vi "Bank Connection Page.vi"(8 "error in (no error)":errorcluster, 11 "Node Ptr":T1 format="%.0x") -> (0 "error out":errorcluster)   [LabVIEW 2011, in "NI 272x Resistive Simulation Custom Device Configuration.lvlib"]
uses:
  NI 272x Resistive Simulation Custom Device Configuration.lvlib
  <vilib>/NI Veristand/Custom Device API/Custom Device Item Ref.ctl
  Globals/Names.vi
  <vilib>/NI Veristand/Custom Device API/Get Item Property (I32).vi
  <vilib>/NI Veristand/Custom Device API/Set Item Property (I32).vi
  <vilib>/NI Veristand/Custom Device API/Custom Device API.lvlib
  NI 272x Resistive Simulation Custom Device Shared.lvlib
panel:
  out "Adjacent Channel #":i32
  in  "Default Value":dbl
  in  "Channel #":i32 min=0
  in  "Header":cluster{"Section Name":string}={"Section Name"="Bank Connection Setting"}
  in  "Description":string
  in  "Name":string
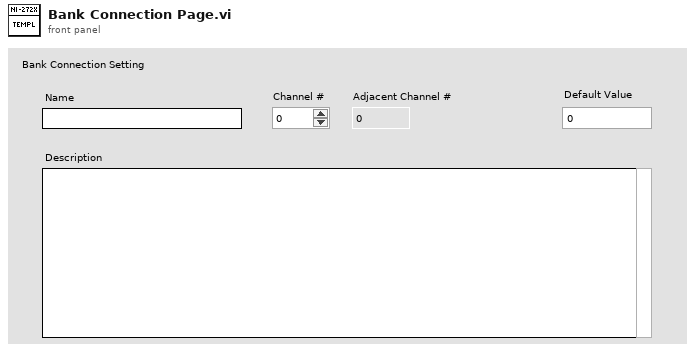
[diagram p1: front panel]
types:
  T1 = typedef "Custom Device API.lvlib/Custom Device Item Ref.ctl" = u64
  T2 = typedef "Custom Device API.lvlib/Custom Device Channel.ctl" = cluster{"Type":T3, "Units":string, "Default Value":dbl, "Faultable":bool, "Scalable":bool}
  T3 = typedef "Custom Device API.lvlib/Custom Device Channel Type.ctl" = enum16{"Input", "Output"}
  T4 = typedef "Custom Device API.lvlib/Custom Device Item Info.ctl" = cluster{"Name":string, "Is Channel":bool, "GUID":string}
  T5 = typedef "Custom Device API.lvlib/Custom Device Commands.ctl" = enum16{"Default", "Item renamed", "Shutdown", "Dynamic button pressed"}
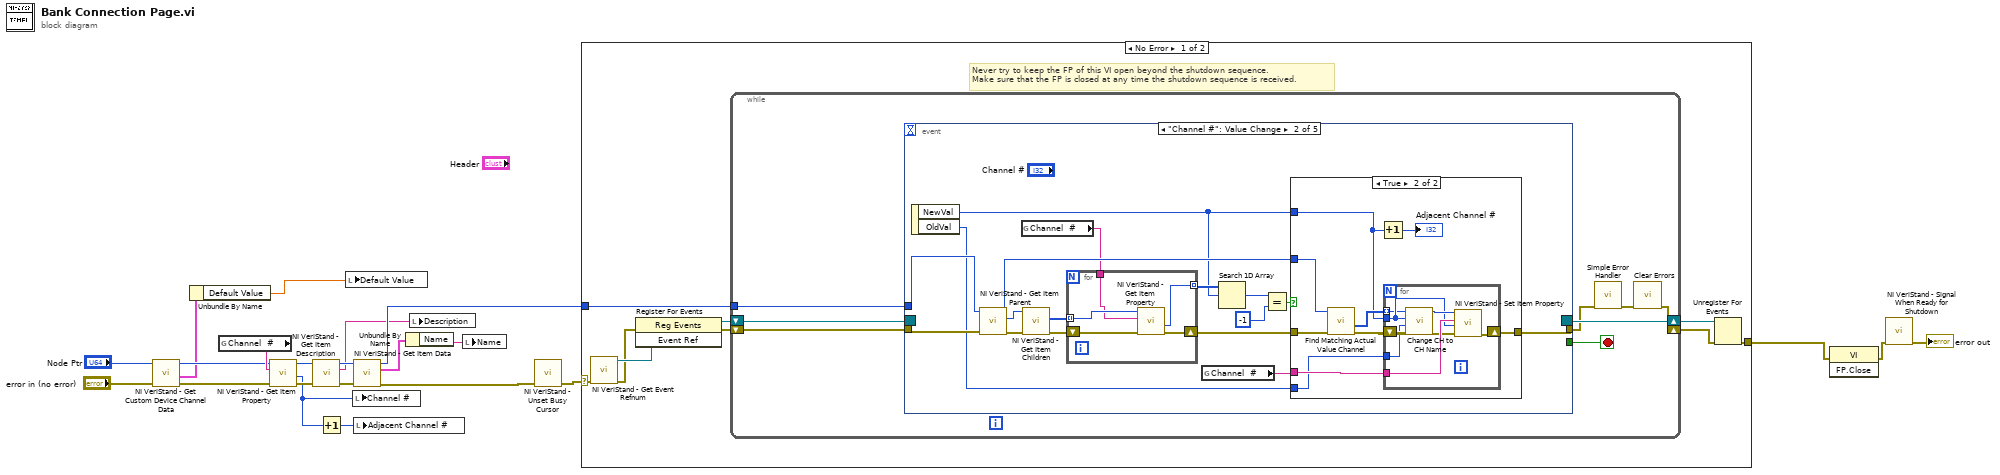
[diagram p0: block diagram]
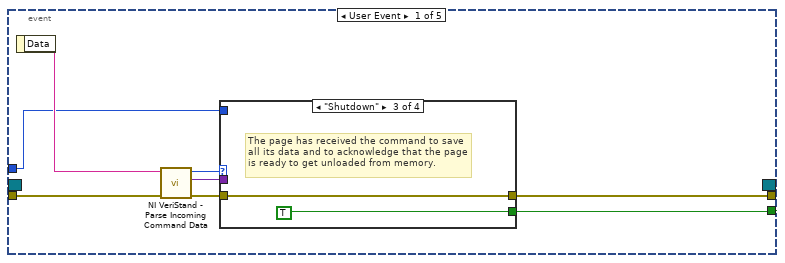
[diagram p2: hidden frame]
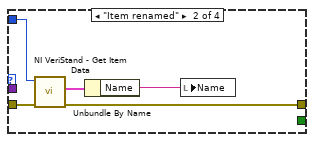
[diagram p4: hidden frame]
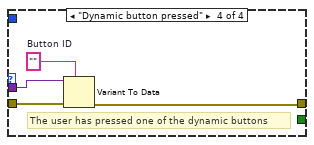
[diagram p5: hidden frame]
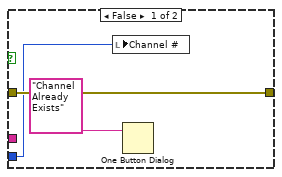
[diagram p6: hidden frame]
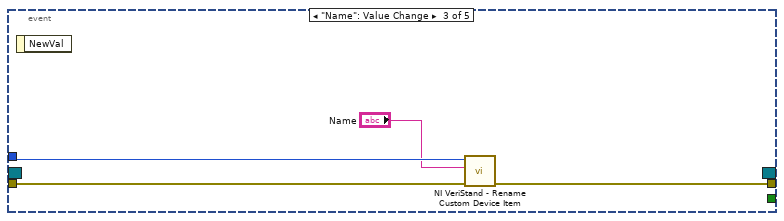
[diagram p7: hidden frame]
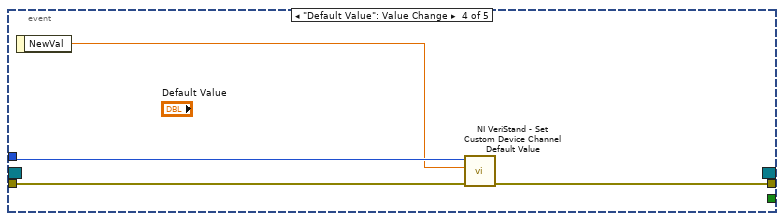
[diagram p8: hidden frame]
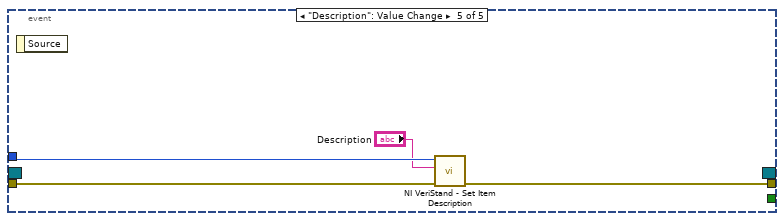
[diagram p9: hidden frame]
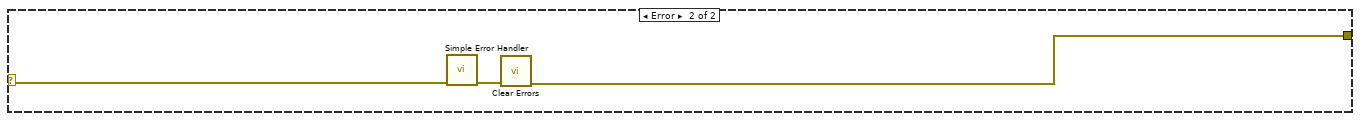
[diagram p10: hidden frame]
diagram:
  n1 = call <vilib>:"NI VeriStand - Get Custom Device Channel Data.vi"("error in (no error)"="error in (no error)", "Channel Ref in"="Node Ptr") -> ("error out"=w5:errorcluster, "Channel"=w2:T2, "Channel Ref out"=w3:T1)  [unwired: 4 in, 3 out]
  n2 = Unbundle By Name(w2) -> ("Default Value"=w1:dbl)
  n3 = global read "Names.vi" "Channel  #"() -> (w9:string)
  n4 = call-poly <vilib>:"NI VeriStand - Get Item Property.vi"("error in (no error)"=w5, "Property Name"=w9, "Item Ref in"=w3) -> ("error out"=w10:errorcluster, "Value"=w7:i32, "Item Ref out"=w11:T1)  [unwired: 5 in, 1 out]
  n5 = call <vilib>:"NI VeriStand - Get Item Description.vi"("error in (no error)"=w10, "Item Ref in"=w11) -> ("error out"=w14:errorcluster, "Description"=w15:string, "Item Ref out"=w16:T1)  [unwired: 7 out]
  n6 = Increment(x=w7) -> (x+1=w6:i32)
  n7 = local write "Default Value"(w1) -> ()
  n8 = local write "Channel #"(w7) -> ()
  n9 = call <vilib>:"NI VeriStand - Get Item Data.vi"("error in (no error)"=w14, "Item Ref in"=w16) -> ("error out"=w8:errorcluster, "Item Info"=w13:T4, "Item Ref out"=w18:T1)  [unwired: 7 out]
  n10 = local write "Adjacent Channel #"(w6) -> ()
  n11 = Unbundle By Name(w13) -> ("Name"=w12:string)
  n12 = local write "Description"(w15) -> ()
  n13 = local write "Name"(w12) -> ()
  n14 = call <vilib>:"NI VeriStand - Unset Busy Cursor.vi"("error in (no error)"=w8) -> ("error out"=w19:errorcluster)  [unwired: 10 out]
  n15 = case shown="No Error" w19 {
    selector: w19 -> [w24 w116]
    tunnel: [w29 w114] -> w22
    tunnel: w18 -> [w25 _]
    frame No Error {
      # "Never try to keep the FP of this VI open beyond the shutdown sequence.\nMake sure that the FP is closed at any time the shutdown sequence is received."
      n16 = call <vilib>:"NI VeriStand - Get Event Refnum.vi"("error in (no error)"=w24) -> ("error out"=w23:errorcluster, "Event Ref"=w28:refnum<user-event>)  [unwired: 9 out]
      n17 = register-events(error in=w23, w28) -> (reference out=w26:refnum<event-registration>, error out=w27:errorcluster)  [unwired: 1 in]
      n18 = while {
        tunnel: w25 -> [w35]
        shift-right: [w33] -> w30
        shift-left: w27 -> [w38]
        shift-right: [w39] -> w31
        shift-left: w26 -> [w37]
        stop <- w36 stop-if-true
        n19 = event shown="[1] \"Channel #\": Value Change" {
          selector: w37 -> [_ _ _ _ _]
          dyn-events: [_ _ _ _ _] -> w39
          timeout: _ -> [_ _ _ _ _]
          tunnel: w38 -> [w47 w66 w105 w109 w112]
          tunnel: [w43 _ _ _ _] -> w36
          tunnel: [w42 w62 w102 w107 w111] -> w32
          tunnel: w35 -> [w41 w65 w104 w108 w113]
          event User Event {
            n20 = event-data() -> ("Data"=w46:string)  [unwired: 1 out]
            n21 = call <vilib>:"NI VeriStand - Parse Incoming Command Data.vi"("error in (no error)"=w47, "Incoming data"=w46) -> ("error out"=w45:errorcluster, "Outgoing data"=w40:variant, "Action"=w44:T5)  [unwired: 7 out]
            n22 = case shown="\"Shutdown\"" w44 {
              tunnel: w45 -> [w48 w53 w54 w59]
              tunnel: [_ _ TRUE _] -> w43
              tunnel: [w48 w50 w54 w56] -> w42
              tunnel: w41 -> [_ w52 _ _]
              tunnel: w40 -> [_ _ _ w58]
              frame "Default", Default {
              }
              frame "Item renamed" {
                n23 = call <vilib>:"NI VeriStand - Get Item Data.vi"("error in (no error)"=w53, "Item Ref in"=w52) -> ("error out"=w50:errorcluster, "Item Info"=w51:T4)  [unwired: 8 out]
                n24 = Unbundle By Name(w51) -> ("Name"=w49:string)
                n25 = local write "Name"(w49) -> ()
              }
              frame "Shutdown" {
                # "The page has received the command to save all its data and to acknowledge that the page is ready to get unloaded from memory."
              }
              frame "Dynamic button pressed" {
                w57 = ""  # Button ID
                # "The user has pressed one of the dynamic buttons"
                n26 = Variant To Data(error in=w59, type=w57, Variant=w58) -> (error out=w56:errorcluster)  [unwired: 1 out]
              }
            }
          }
          event "Channel #": Value Change {
            n27 = event-data() -> ("NewVal"=w64:i32, "OldVal"=w63:i32)  [unwired: 1 out]
            n28 = call <vilib>:"NI VeriStand - Get Item Parent.vi"("error in (no error)"=w66, "Item Ref in"=w65) -> ("error out"=w67:errorcluster, "Parent Ref"=w68:T1, "Item Ref out"=w76:T1)  [unwired: 6 in, 1 out]
            n29 = global read "Names.vi" "Channel  #"() -> (w60:string)
            n30 = call <vilib>:"NI VeriStand - Get Item Children.vi"("error in (no error)"=w67, "Item Ref in"=w68) -> ("error out"=w70:errorcluster, "Child Refs"=w69:T1[])  [unwired: 6 in, 2 out]
            n31 = for {
              tunnel: w69 -> [w99] mode=indexing
              shift-right: [w100] -> w75
              shift-left: w70 -> [w101]
              tunnel: [w98] -> w71 mode=indexing
              tunnel: w60 -> [w97]
              n32 = call-poly <vilib>:"NI VeriStand - Get Item Property.vi"("error in (no error)"=w101, "Property Name"=w97, "Item Ref in"=w99) -> ("error out"=w100:errorcluster, "Value"=w98:i32)  [unwired: 5 in, 2 out]
            }
            n33 = global read "Names.vi" "Channel  #"() -> (w61:string)
            n34 = Search 1D Array(1D array=w71, element=w64) -> (index of element=w72:i32)  [unwired: 1 in]
            n35 = Equal?(x=w72, y=-1) -> (x = y?=w74:bool)
            n36 = case shown="True" w74 {
              tunnel: w75 -> [w79 w86]
              tunnel: w76 -> [_ w85]
              tunnel: w61 -> [_ w87]
              tunnel: w64 -> [_ w81]
              tunnel: [w79 w88] -> w62
              tunnel: w63 -> [w77 w82]
              frame False {
                n37 = local write "Channel #"(w77) -> ()
                n38 = One Button Dialog(message="Channel Already Exists") -> ()  [unwired: 1 in, 1 out]
              }
              frame True {
                n39 = call "Find Matching Actual Value Channel.vi"("error in (no error)"=w86, "Desired item ref in"=w85) -> ("error out"=w84:errorcluster, "Both refs"=w83:T1[])  [unwired: 5 in, 3 out]
                n40 = Increment(x=w81) -> (x+1=→"Adjacent Channel #":i32)
                n41 = for {
                  tunnel: w87 -> [w95]
                  shift-right: [w96] -> w88
                  shift-left: w84 -> [w93]
                  tunnel: w81 -> [w91]
                  tunnel: w83 -> [w90] mode=indexing
                  tunnel: w82 -> [w89]
                  n42 = call "Change CH to CH Name.vi"("error in (no error)"=w93, "Old #"=w89, "New #"=w91, "Node Ptr"=w90) -> ("error out"=w94:errorcluster, "Node Ptr out"=w92:T1)  [unwired: 6 in]
                  n43 = call-poly <vilib>:"NI VeriStand - Set Item Property.vi"("error in (no error)"=w94, "Value"=w91, "Property Name"=w95, "Item Ref in"=w92) -> ("error out"=w96:errorcluster)  [unwired: 5 in, 2 out]
                }
              }
            }
          }
          event "Name": Value Change {
            n44 = event-data() -> ()  [unwired: 2 out]
            n45 = call <vilib>:"NI VeriStand - Rename Custom Device Item.vi"("error in (no error)"=w105, "New Name"="Name", "Item Ref in"=w104) -> ("error out"=w102:errorcluster)  [unwired: 8 out]
          }
          event "Default Value": Value Change {
            n46 = event-data() -> ("NewVal"=w106:dbl)  [unwired: 1 out]
            n47 = call <vilib>:"NI VeriStand - Set Custom Device Channel Default Value.vi"("error in (no error)"=w109, "Default Value"=w106, "Channel Ref in"=w108) -> ("error out"=w107:errorcluster)  [unwired: 7 in, 1 out]
          }
          event "Description": Value Change {
            n48 = event-data() -> ()  [unwired: 2 out]
            n49 = call <vilib>:"NI VeriStand - Set Item Description.vi"("error in (no error)"=w112, "Description"="Description", "Item Ref in"=w113) -> ("error out"=w111:errorcluster)  [unwired: 8 out]
          }
        }
        n50 = call <vilib>:"Simple Error Handler.vi"("error in (no error)"=w32) -> ("error out"=w34:errorcluster)  [unwired: 1 in, 7 out]
        n51 = call <vilib>:"Clear Errors.vi"("error in (no error)"=w34) -> ("error out"=w33:errorcluster)  [unwired: 6 out]
      }
      n52 = Unregister For Events(event registration refnum=w31, error in=w30) -> (error out=w29:errorcluster)
    }
    frame Error {
      n53 = call <vilib>:"Simple Error Handler.vi"("error in (no error)"=w116) -> ("error out"=w115:errorcluster)  [unwired: 1 in, 7 out]
      n54 = call <vilib>:"Clear Errors.vi"("error in (no error)"=w115) -> ("error out"=w114:errorcluster)  [unwired: 6 out]
    }
  }
  n55 = invoke class="VI" method="FP.Close"(error in=w22) -> (error out=w21:errorcluster)  [unwired: 2 in, 2 out]
  n56 = call <vilib>:"NI VeriStand - Signal When Ready for Shutdown.vi"("error in (no error)"=w21) -> ("error out"=→"error out":errorcluster)  [unwired: 10 out]
